vi "Expanded Terminals.vi"(9 "State":T10, 10 "Sizes":T1) -> (3 "Terms":T2)   [LabVIEW 2020, in "FlexBlock.xnode"]
uses:
  FlexBlock.xnode
  State.ctl
  FlexBlocks/Type Descriptor.ctl
  FlexBlocks/Terminal Direction.ctl
  FlexBlocks/Value Mode.ctl
  FlexBlocks/Terminal State.ctl
  FlexBlocks/Special Terminal.ctl
  FlexBlocks/Errors.ctl
  <vilib>/picture/picture.llb/imagedata.ctl
  FlexBlocks/Calculated Sizes.ctl
  <vilib>/XNodeSupport/XNodeTerm4Array.ctl
  <vilib>/XNodeSupport/XNodeTerm4.ctl
  <vilib>/XNodeSupport/XNodeString.ctl
  <vilib>/XNodeSupport/XNodeVariant.ctl
  <vilib>/XNodeSupport/XNodeRect32.ctl
  <vilib>/XNodeSupport/XNodeInt.ctl
  <vilib>/XNodeSupport/XNodeBool.ctl
  <vilib>/XNodeSupport/XNodeTermDirection.ctl
  FlexBlocks/Size Constants.ctl
  FlexBlocks/FlexBlocks.lvlib
  <vilib>/XNodeSupport/NI_XNodeSupport.lvlib
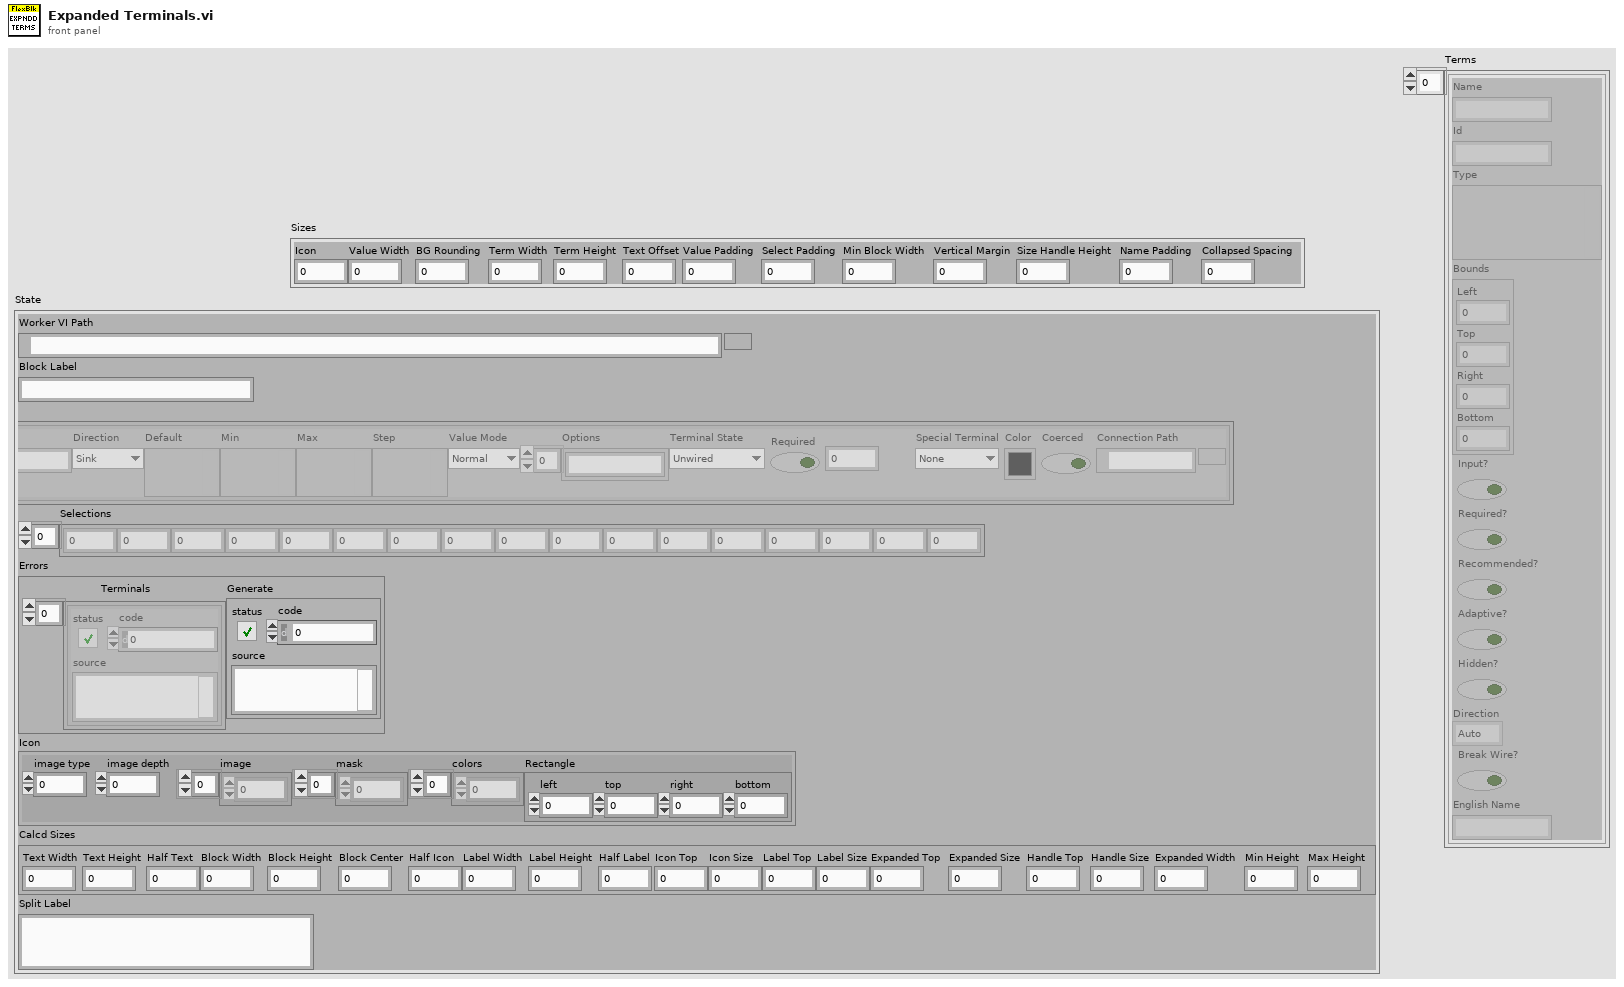
[diagram p1: front panel]
types:
  T1 = typedef "FlexBlocks.lvlib/Size Constants.ctl" = cluster{"Icon":i32, "Value Width":i32, "BG Rounding":i32, "Term Width":i32, "Term Height":i32, "Text Offset":i32, "Value Padding":i32, "Select Padding":i32, "Min Block Width":i32, "Vertical Margin":i32, "Size Handle Height":i32, "Name Padding":i32, "Collapsed Spacing":i32}
  T2 = typedef "NI_XNodeSupport.lvlib/XNodeTerm4Array.ctl" = T3[]
  T3 = typedef "NI_XNodeSupport.lvlib/XNodeTerm4.ctl" = cluster{"Name":T4, "Id":T4, "Type":T5, "Bounds":T6, "Input?":T8, "Required?":T8, "Recommended?":T8, "Adaptive?":T8, "Hidden?":T8, "Direction":T9, "Break Wire?":T8, "English Name":T4}
  T4 = typedef "NI_XNodeSupport.lvlib/XNodeString.ctl" = string
  T5 = typedef "NI_XNodeSupport.lvlib/XNodeVariant.ctl" = variant
  T6 = typedef "NI_XNodeSupport.lvlib/XNodeRect32.ctl" = cluster{"Left":T7, "Top":T7, "Right":T7, "Bottom":T7}
  T7 = typedef "NI_XNodeSupport.lvlib/XNodeInt.ctl" = i32
  T8 = typedef "NI_XNodeSupport.lvlib/XNodeBool.ctl" = bool
  T9 = typedef "NI_XNodeSupport.lvlib/XNodeTermDirection.ctl" = enum32{"Auto", "Up", "Down", "Left", "Right", "Center"}
  T10 = typedef "FlexBlock.xnode/State.ctl" = cluster{"Worker VI Path":path, "Block Label":string, "Types":T11[], "Selections":i32[], "Errors":T16, "Icon":T17, "Calcd Sizes":T18, "Split Label":string}
  T11 = typedef "FlexBlocks.lvlib/Type Descriptor.ctl" = cluster{"Name":string, "Direction":T12, "Default":variant, "Min":variant, "Max":variant, "Step":variant, "Value Mode":T13, "Options":string[], "Terminal State":T14, "Required":bool, "Connpane Index":i32, "Special Terminal":T15, "Color":u32, "Coerced":bool, "Connection Path":path}
  T12 = typedef "FlexBlocks.lvlib/Terminal Direction.ctl" = enum16{"Sink", "Source"}
  T13 = typedef "FlexBlocks.lvlib/Value Mode.ctl" = enum16{"Normal", "Range", "Select"}
  T14 = typedef "FlexBlocks.lvlib/Terminal State.ctl" = enum16{"Unwired", "BadType", "BadRef", "Channel", "Value", "Control Ref"}
  T15 = typedef "FlexBlocks.lvlib/Special Terminal.ctl" = enum16{"None", "Action", "Init", "Tag", "State in", "State out", "Error"}
  T16 = typedef "FlexBlocks.lvlib/Errors.ctl" = cluster{"Terminals":errorcluster[], "Generate":errorcluster}
  T17 = typedef "imagedata.ctl" = cluster{"image type":i32, "image depth":i32, "image":u8[], "mask":u8[], "colors":u32[], "Rectangle":cluster{"left":i16, "top":i16, "right":i16, "bottom":i16}}
  T18 = typedef "FlexBlocks.lvlib/Calculated Sizes.ctl" = cluster{"Text Width":i32, "Text Height":i32, "Half Text":i32, "Block Width":i32, "Block Height":i32, "Block Center":i32, "Half Icon":i32, "Label Width":i32, "Label Height":i32, "Half Label":i32, "Icon Top":i32, "Icon Size":i32, "Label Top":i32, "Label Size":i32, "Expanded Top":i32, "Expanded Size":i32, "Handle Top":i32, "Handle Size":i32, "Expanded Width":i32, "Min Height":i32, "Max Height":i32}
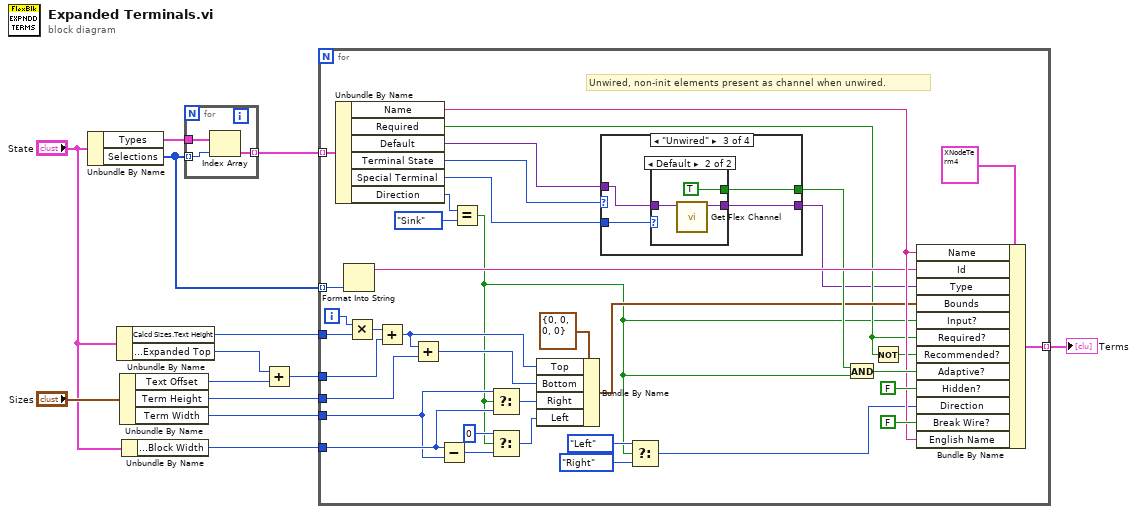
[diagram p0: block diagram]
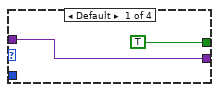
[diagram p2: hidden frame]
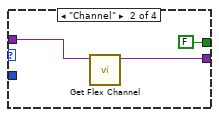
[diagram p3: hidden frame]
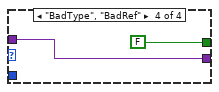
[diagram p5: hidden frame]
diagram:
  n1 = Unbundle By Name("State") -> ("Types"=w13:T11[], "Selections"=w12:i32[])
  n2 = Unbundle By Name("State") -> ("Calcd Sizes.Text Height"=w8:i32, "Calcd Sizes.Expanded Top"=w2:i32)
  n3 = Unbundle By Name("Sizes") -> ("Text Offset"=w6:i32, "Term Height"=w7:i32, "Term Width"=w3:i32)
  n4 = Unbundle By Name("State") -> ("Calcd Sizes.Block Width"=w4:i32)
  n5 = for {
    tunnel: w13 -> [w16]
    tunnel: w12 -> [w15] mode=indexing
    tunnel: [w14] -> w11 mode=indexing
    n6 = Index Array(array=w16, index=w15) -> (element=w14:T11)
  }
  n7 = Add(x=w2, y=w6) -> (x+y=w1:i32)
  n8 = for {
    tunnel: w12 -> [w41] mode=indexing
    tunnel: w11 -> [w53] mode=indexing
    tunnel: [w42] -> w10 mode=indexing
    tunnel: w8 -> [w36]
    tunnel: w7 -> [w30]
    tunnel: w1 -> [w31]
    tunnel: w4 -> [w25]
    tunnel: w3 -> [w24]
    i -> [w35]
    # "Unwired, non-init elements present as channel when unwired."
    n9 = Unbundle By Name(w53) -> ("Name"=w44:string, "Required"=w21:bool, "Default"=w20:variant, "Terminal State"=w38:T14, "Special Terminal"=w17:T15, "Direction"=w52:T12)
    n10 = Format Into String(w41) -> (resulting string=w40:string)  [unwired: 3 in, 1 out]
    n11 = Multiply(x=w35, y=w36) -> (x*y=w32:i32)
    n12 = Add(x=w32, y=w31) -> (x+y=w22:i32)
    n13 = Add(x=w22, y=w30) -> (x+y=w29:i32)
    n14 = Subtract(x=w25, y=w24) -> (x-y=w28:i32)
    n15 = Equal?(x=w52, y=Terminal_Direction."Sink") -> (x = y?=w18:bool)
    n16 = Select(t=w24, s=w18, f=w25) -> (s? t:f=w23:i32)
    n17 = Select(t=0, s=w18, f=w28) -> (s? t:f=w26:i32)
    n18 = Bundle By Name(cluster=T6 {"Left"=0, "Top"=0, "Right"=0, "Bottom"=0} ("Bounds"), "Top"=w22, "Bottom"=w29, "Right"=w23, "Left"=w26) -> (w33:T6)
    n19 = case shown="\"Unwired\"" w38 {
      tunnel: [TRUE FALSE w59 FALSE] -> w37
      tunnel: w20 -> [w54 w57 w62 w67]
      tunnel: [w54 w56 w61 w67] -> w19
      tunnel: w17 -> [_ _ w60 _]
      frame Default {
      }
      frame "Channel" {
        n20 = call "Get Flex Channel.vi"("Element Type"=w57) -> ("Data Type"=w56:variant)  [unwired: 10 in]
      }
      frame "Unwired" {
        n21 = case shown="Default" w60 {
          tunnel: w62 -> [w63 w66]
          tunnel: [w63 w65] -> w61
          tunnel: [_ TRUE] -> w59
          frame "Init" {
          }
          frame Default {
            n22 = call "Get Flex Channel.vi"("Element Type"=w66) -> ("Data Type"=w65:variant)  [unwired: 10 in]
          }
        }
      }
      frame "BadType", "BadRef" {
      }
    }
    n23 = Select(t=XNodeTermDirection."Left" ("Direction"), s=w18, f=XNodeTermDirection."Right" ("Direction")) -> (s? t:f=w43:T9)
    n24 = And(x=w37, y=w18) -> (x .and. y?=w45:bool)
    n25 = Not(x=w21) -> (.not. x?=w39:bool)
    n26 = Bundle By Name(cluster=T3 {"Name"="", "Id"="", "Type"=variant, "Bounds"={"Left"=0, "Top"=0, "Right"=0, "Bottom"=0}, "Input?"=FALSE, "Required?"=FALSE, "Recommended?"=FALSE, "Adaptive?"=FALSE, "Hidden?"=FALSE, "Direction"=enum."Auto", "Break Wire?"=FALSE, "English Name"=""} ("Term 4"), "Name"=w44, "Id"=w40, "Type"=w19, "Bounds"=w33, "Input?"=w18, "Required?"=w21, "Recommended?"=w39, "Adaptive?"=w45, "Hidden?"=T8 FALSE, "Direction"=w43, "Break Wire?"=T8 FALSE, "English Name"=w44) -> (w42:T3)
  }
  "Terms" <- w10
